vi "ParameterInterceptorInfo.vi"(0 "Data name":string) -> (1 "arrayLevel":i32, 2 "interceptorVI":path, 3 "get?":bool, 4 "intercept?":bool)   [LabVIEW 2013]
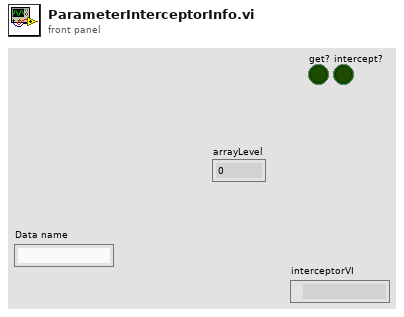
[diagram p1: front panel]
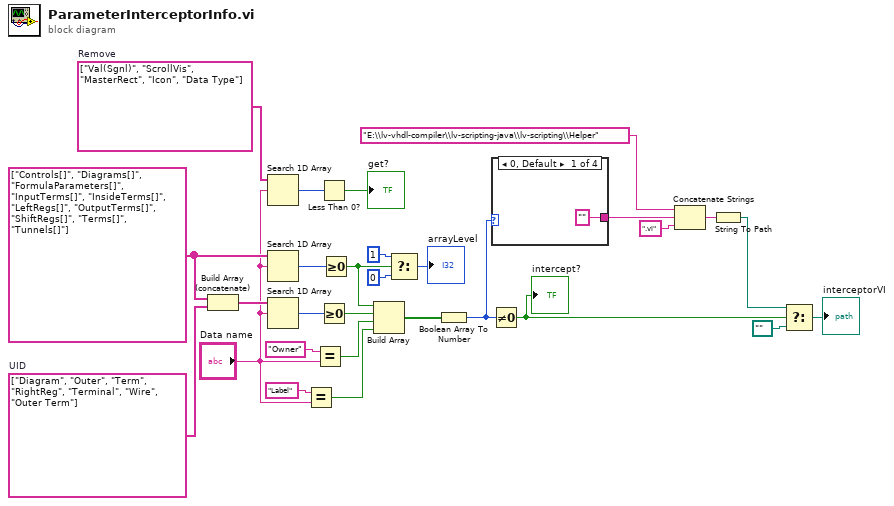
[diagram p0: block diagram]
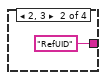
[diagram p2: hidden frame]
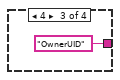
[diagram p3: hidden frame]
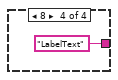
[diagram p4: hidden frame]
diagram:
  w19 = string[] ["Val(Sgnl)", "ScrollVis", "MasterRect", "Icon", "Data Type"]  # Remove
  w17 = string[] ["Diagram", "Outer", "Term", "RightReg", "Terminal", "Wire", "Outer Term"]  # UID
  w18 = string[] ["Controls[]", "Diagrams[]", "FormulaParameters[]", "InputTerms[]", "InsideTerms[]", "LeftRegs[]", "OutputTerms[]", "ShiftRegs[]", "Terms[]", "Tunnels[]"]
  n1 = Build Array (concatenate)(w18, w17) -> (w16:string[])
  n2 = Search 1D Array(1D array=w19, element="Data name") -> (index of element=w20:i32)  [unwired: 1 in]
  n3 = Search 1D Array(1D array=w18, element="Data name") -> (index of element=w28:i32)  [unwired: 1 in]
  n4 = Search 1D Array(1D array=w16, element="Data name") -> (index of element=w24:i32)  [unwired: 1 in]
  n5 = Equal?(x="Label" ("Remove"), y="Data name") -> (x = y?=w11:bool)
  n6 = Equal?(x="Owner" ("Remove"), y="Data name") -> (x = y?=w14:bool)
  n7 = Less Than 0?(x=w20) -> (x < 0?=→"get?":bool)
  n8 = Greater Or Equal To 0?(x=w24) -> (x >= 0?=w22:bool)
  n9 = Greater Or Equal To 0?(x=w28) -> (x >= 0?=w23:bool)
  n10 = Build Array(w23, w22, w14, w11) -> (w21:bool[])
  n11 = Select(t=1, s=w23, f=0) -> (s? t:f=→"arrayLevel":i32)
  n12 = Boolean Array To Number(Boolean array=w21) -> (number=w6:u32)
  n13 = Not Equal To 0?(x=w6) -> (x != 0?=w4:bool)
  "intercept?" <- w4
  n14 = case shown="0, Default" w6 {
    tunnel: ["" "RefUID" "OwnerUID" "LabelText"] -> w7
    frame 0, Default {
    }
    frame 2, 3 {
    }
    frame 4 {
    }
    frame 8 {
    }
  }
  n15 = Concatenate Strings("E:\\lv-vhdl-compiler\\lv-scripting-java\\lv-scripting\\Helper" ("Directory"), w7, ".vi" ("string")) -> (w9:string)
  n16 = String To Path(string=w9) -> (path=w2:path)
  n17 = Select(t=w2, s=w4, f=path "") -> (s? t:f=→"interceptorVI":path)
